vi "get Data.vi"(0 "identifier":string, 1 "spectra_size":u32, 2 "stats":T2, 5 "Board":u16, 7 "id":u32, 9 "values":u64[](array[numeric]), 11 "error in (no error)":errorcluster) -> (3 "spectra_size out":u32, 4 "function return":bool, 10 "values out":u64[](array[numeric]), 13 "stats out":T1, 15 "error out":errorcluster)   [LabVIEW 2015, in "XGL_DPP.lvlib"]
doc: "EXTERN DECLSPEC bool CALL_CONV getAllData(const char* identifier,\n unsigned short Board,\n unsigned short int* values,\n unsigned long int* id,\n double* stats,\n unsigned long long int* advstats,\n unsigned int& spectra_size,\n unsigned int& data_number,\n unsigned short int& acq_status\n);"
uses:
  XGL_DPP.lvlib
  XGL_DPP.dll
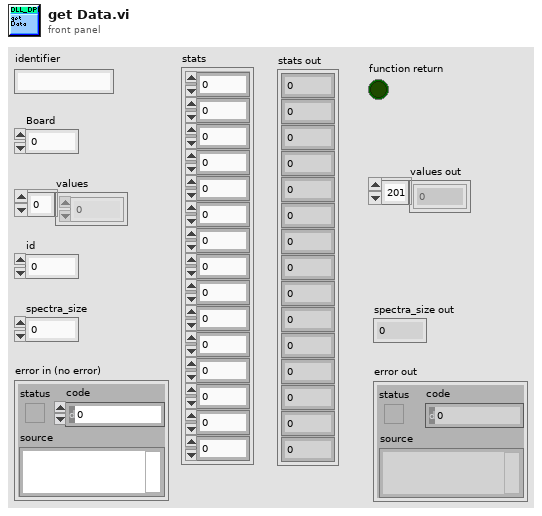
[diagram p1: front panel]
types:
  T1 = cluster{u64, u64, dbl, dbl, u32, u32, u32, u32, u32, u32, u32, u32, u32, u32, u32}
  T2 = cluster{u64, u64, dbl, dbl, u64, u32, u32, u32, u32, u32, u32, u32, u32, u32, u32}
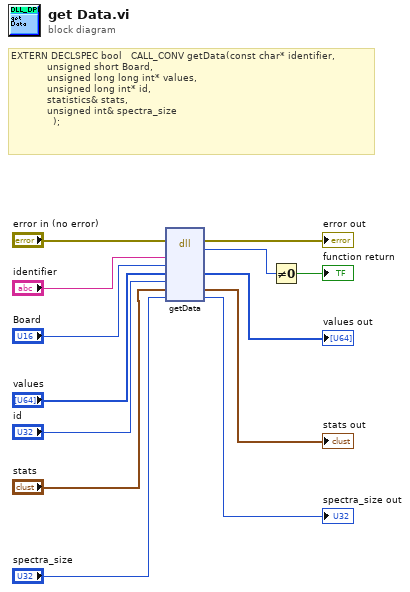
[diagram p0: block diagram]
diagram:
  # "EXTERN DECLSPEC bool   CALL_CONV getData(const char* identifier,\n\t\t\t\t\t\t\t\t\t\t\t\tunsigned short Board,\n\t\t\t\t\t\t\t\t\t\t\t\tunsigned long long int* values,\n\t\t\t\t\t\t\t\t\t\t\t\tunsigned long int* id,\n\t\t\t\t\t\t\t\t\t\t\t\tstatistics& stats,\n\t\t\t\t\t\t\t\t\t\t\t\tunsigned int& spectra_size\n\t\t\t\t\t\t\t\t\t\t\t   );"
  n1 = dll-call lib="D:/Users/XRF/Desktop/Dante_acquire4/libs/Dante/XGL_DPP.*" fn="getData"(error in="error in (no error)", "identifier"="identifier", "Board"="Board", "values"="values", "id"="id", "stats"="stats", "spectra_size"="spectra_size") -> (error out=→"error out":errorcluster, "return type"=w12:u8, "values"=→"values out":u64[], "stats"=→"stats out":T2, "spectra_size"=→"spectra_size out":u32)  [unwired: 5 in, 1 out]
  n2 = Not Equal To 0?(x=w12) -> (x != 0?=→"function return":bool)
